vi "AF_ConfigurationMemory.vi"(1 "AF_MessaageWireConfiguration":T2={"Edge thickness"=1, "Edge color"=5667411, "Center thickness"=1, "Center pattern"=enum."Solid", "CenterColor1"=9740924, "CenterColor2"=8694662, "Tunnels and terminals colors"=131187}, 2 "Icon":string="bluefull.png", 3 "AF_Settings":T1, 5 "error in (no error)":errorcluster, 6 "Action":enum16{"Read", "Load", "Save", "Set"}(ring)) -> (15 "AF_MessaageWireConfigurationOut":T2={"Edge thickness"=1, "Edge color"=5667411, "Center thickness"=1, "Center pattern"=enum."Solid", "CenterColor1"=9740924, "CenterColor2"=8694662, "Tunnels and terminals colors"=131187}, 16 "IconOut":string="bluefull.png", 17 "AF_SettingsOut":T1, 19 "error out":errorcluster)   [LabVIEW 2014]
uses:
  <resource>/Framework/Providers/Open_GDS/SubVIs/GOOP_WireConfigurationType.ctl
  <resource>/Framework/Providers/Open_GDS/SubVIs/GOOP_WirePattern.ctl
  <resource>/Framework/Providers/Open_GDS/ClassProviders/Common/AF/AF_SettingsType.ctl
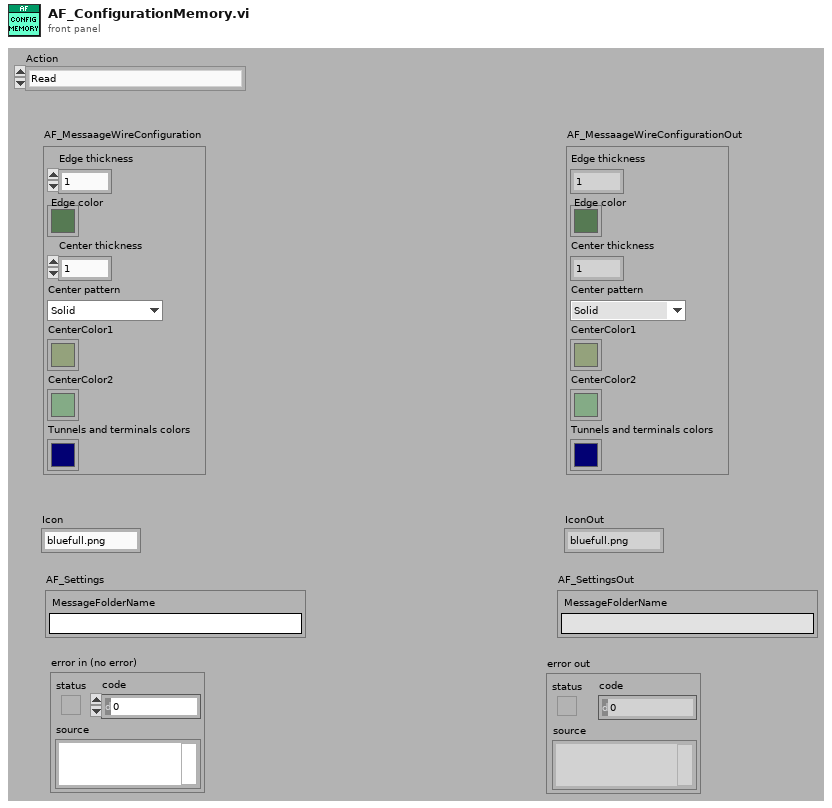
[diagram p1: front panel]
types:
  T1 = typedef "AF_SettingsType.ctl" = cluster{"MessageFolderName":string}
  T2 = typedef "GOOP_WireConfigurationType.ctl" = cluster{"Edge thickness":i32, "Edge color":u32, "Center thickness":i32, "Center pattern":T3, "CenterColor1":u32, "CenterColor2":u32, "Tunnels and terminals colors":u32}
  T3 = typedef "GOOP_WirePattern.ctl" = enum16{"Solid", "Large dash", "Small dash"}
  T4 = cluster{"WireConfiguration":T2, "Icon":string, "AF_Settings":T1}
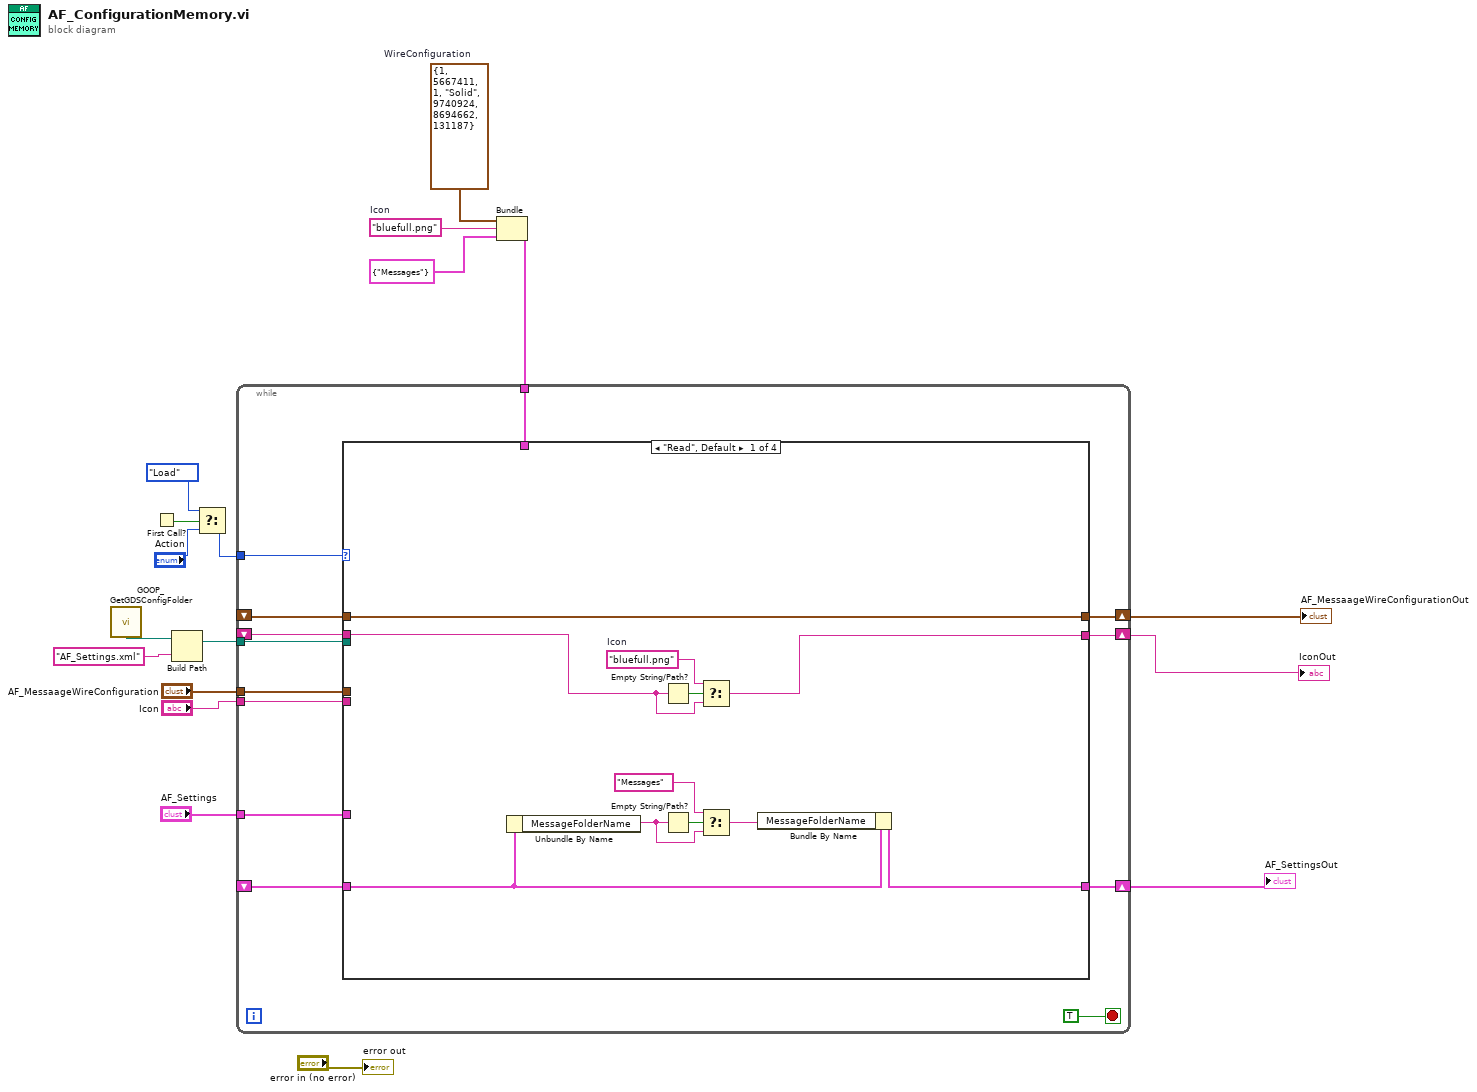
[diagram p0: block diagram]
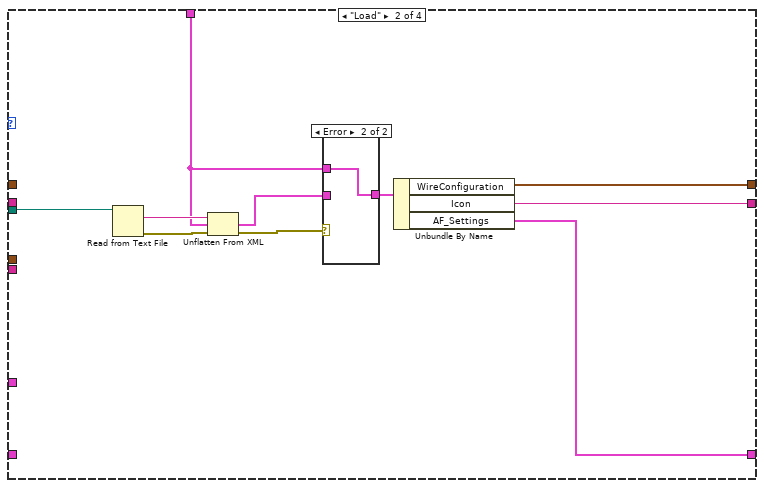
[diagram p2: hidden frame]
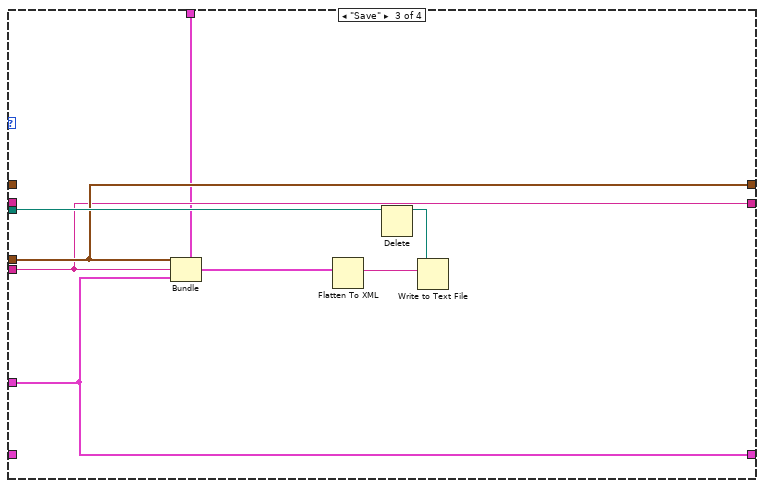
[diagram p4: hidden frame]
diagram:
  w14 = "bluefull.png"  # Icon
  w15 = T2 {"Edge thickness"=1, "Edge color"=5667411, "Center thickness"=1, "Center pattern"=enum."Solid", "CenterColor1"=9740924, "CenterColor2"=8694662, "Tunnels and terminals colors"=131187}  # WireConfiguration
  n1 = call <resource>:"GOOP_GetGDSConfigFolder.vi"() -> ("GDSFolderPath"=w17:path)
  n2 = First Call?() -> (First Call?: T/F=w10:bool)
  n3 = Build Path(base path=w17, name or relative path="AF_Settings.xml") -> (appended path=w16:path)
  n4 = Select(t=enum16{"Read", "Load", "Save", "Set"}."Load", s=w10, f="Action") -> (s? t:f=w8:enum16{"Read", "Load", "Save", "Set"})
  n5 = Bundle("WireConfiguration"=w15, "Icon"=w14, "AF_Settings"=T1 {"MessageFolderName"="Messages"}) -> (w13:T4)  [unwired: 1 in]
  n6 = while {
    tunnel: w8 -> [w31]
    tunnel: w16 -> [w30]
    tunnel: w13 -> [w29]
    shift-right: [w27] -> w12
    shift-left: _ -> [w25]
    shift-right: [w26] -> w11
    shift-left: _ -> [w24]
    tunnel: "AF_MessaageWireConfiguration" -> [w23]
    tunnel: "Icon" -> [w22]
    shift-right: [w21] -> w1
    shift-left: _ -> [w20]
    tunnel: "AF_Settings" -> [w19]
    stop <- TRUE stop-if-true
    n7 = case shown="\"Read\", Default" w31 {
      tunnel: w30 -> [_ w47 w60 _]
      tunnel: w29 -> [_ w46 w56 _]
      tunnel: [w42 w45 w58 w65] -> w27
      tunnel: [w32 w44 w57 w64] -> w26
      tunnel: w25 -> [w42 _ _ _]
      tunnel: w24 -> [w33 _ _ _]
      tunnel: w23 -> [_ _ w58 w65]
      tunnel: w22 -> [_ _ w57 w64]
      tunnel: [w36 w43 w55 w63] -> w21
      tunnel: w20 -> [w37 _ _ _]
      tunnel: w19 -> [_ _ w55 w63]
      frame "Read", Default {
        w34 = "bluefull.png"  # Icon
        n8 = Unbundle By Name(w37) -> ("MessageFolderName"=w39:string)
        n9 = Empty String/Path?(string/path=w33) -> (empty?=w35:bool)
        n10 = Empty String/Path?(string/path=w39) -> (empty?=w41:bool)
        n11 = Select(t=w34, s=w35, f=w33) -> (s? t:f=w32:string)
        n12 = Select(t="Messages" ("Name"), s=w41, f=w39) -> (s? t:f=w38:string)
        n13 = Bundle By Name(cluster=w37, "MessageFolderName"=w38) -> (w36:T1)
      }
      frame "Load" {
        n14 = Read from Text File(file (use dialog)=w47) -> (text=w48:string, error out=w49:errorcluster)  [unwired: 3 in, 2 out]
        n15 = Unflatten From XML(xml string=w48, type=w46, error in (no error)=w49) -> (value=w51:T4, error out=w50:errorcluster)
        n16 = case shown="Error" w50 {
          tunnel: w51 -> [w53 _]
          tunnel: [w53 w54] -> w52
          tunnel: w46 -> [_ w54]
          frame No Error {
          }
          frame Error {
          }
        }
        n17 = Unbundle By Name(w52) -> ("WireConfiguration"=w45:T2, "Icon"=w44:string, "AF_Settings"=w43:T1)
      }
      frame "Save" {
        n18 = Bundle(cluster=w56, "WireConfiguration"=w58, "Icon"=w57, "AF_Settings"=w55) -> (w59:T4)
        n19 = Flatten To XML(anything=w59) -> (xml string=w61:string)
        n20 = Delete(path (use dialog)=w60) -> (deleted path=w62:path)  [unwired: 4 in, 2 out]
        n21 = Write to Text File(file (use dialog)=w62, text=w61) -> ()  [unwired: 2 in, 3 out]
      }
      frame "Set" {
      }
    }
  }
  "AF_MessaageWireConfigurationOut" <- w12
  "IconOut" <- w11
  "AF_SettingsOut" <- w1
  "error out" <- "error in (no error)"
